vi "HRTF_SynchronizedMeasurement.vi"() -> ()   [LabVIEW 2017]
uses:
  9d5949f9-07ca-45c6-940a-2e3a62ca42df.vi
  <vilib>/express/express analysis/Spectral/Block/exnSpectralBlock spectral measurements RMS poly.vi
  <vilib>/express/express analysis/Spectral/Block/exnSpectralBlock spectral measurements RMS array WFM.vi
  <vilib>/express/express analysis/Spectral/XNode/ExpressSpectralMeasurementsBlockNode.xnode
panel:
  out "current file":dbl
  in  "Number of repetitions (200 is a full revolution)":dbl=200.0
  in  "Rotate stage at COM5":bool=TRUE
  in  "Stim muliplier":dbl=7.0
  in  "4kHz High-pass for stim":bool
  in  "Samples to Read":i32=262144
  in  "Analog Input Sample Clock Source":tag="/Dev1/ao/SampleClock"
  out "Actual Update Generation Rate":dbl=5000.0 format="%0.2f"
  out "Actual Input Rate":dbl=10000.0 format="%0.2f"
  in  "rate":dbl=500000.0 caption="Update Generation Rate" format="%0.2f"
  in  "minimum value":dbl=-10.0 caption="Output Minimum Value" format="%0.2f"
  in  "maximum value":dbl=10.0 caption="Output Maximum Value" format="%0.2f"
  in  "physical channels":tag="Dev1/ao0" caption="Output Physical Channels"
  in  "Maximum Value":dbl=10.0 caption="Input Maximum Value" format="%0.2f"
  in  "Minimum Value":dbl=-10.0 caption="Input Minimum Value" format="%0.2f"
  in  "Rate":dbl=500000.0 caption="Input Rate" format="%0.2f"
  in  "Physical Channel":tag="Dev1/ai0" caption="Input Physical Channel"
  in  "100 Hz high-pass for display":bool
  out "Waveform Graph 2":cluster{"f0":dbl, "df":dbl, "magnitude":dbl[]}[](graph)
  out "Waveform Graph":waveform(dbl)[](graph)
  # "Multiplier was 7 for HRTF measurements.\n4 kHz filter was off for the initial measurement, but it should not affect\nthe response in high frequency.\nIt may not work with 7 V stim."
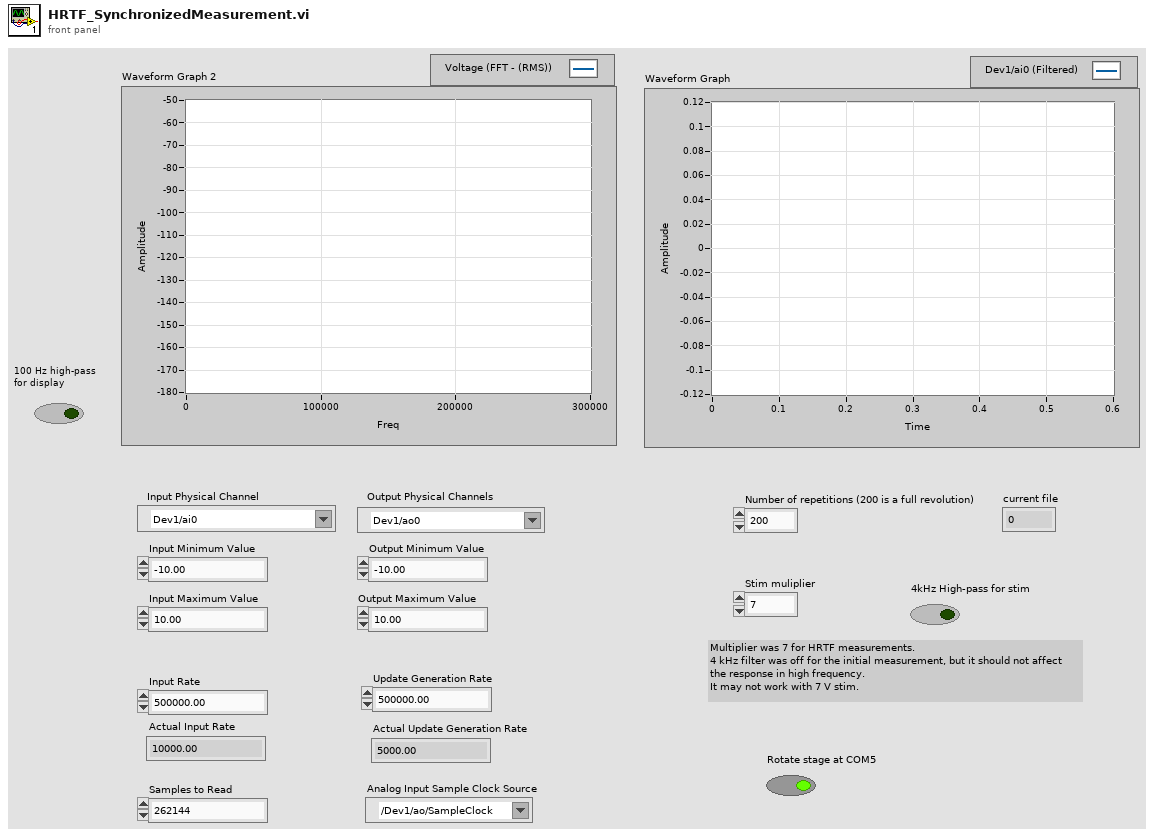
[diagram p1: front panel]
types:
  T1 = cluster{"averaging mode":u16, "weighting mode":u16, "number of averages":u32}
  T2 = cluster{"dB On (F)":bool, "unwrap phase (F)":bool, "convert to degree (F)":bool}
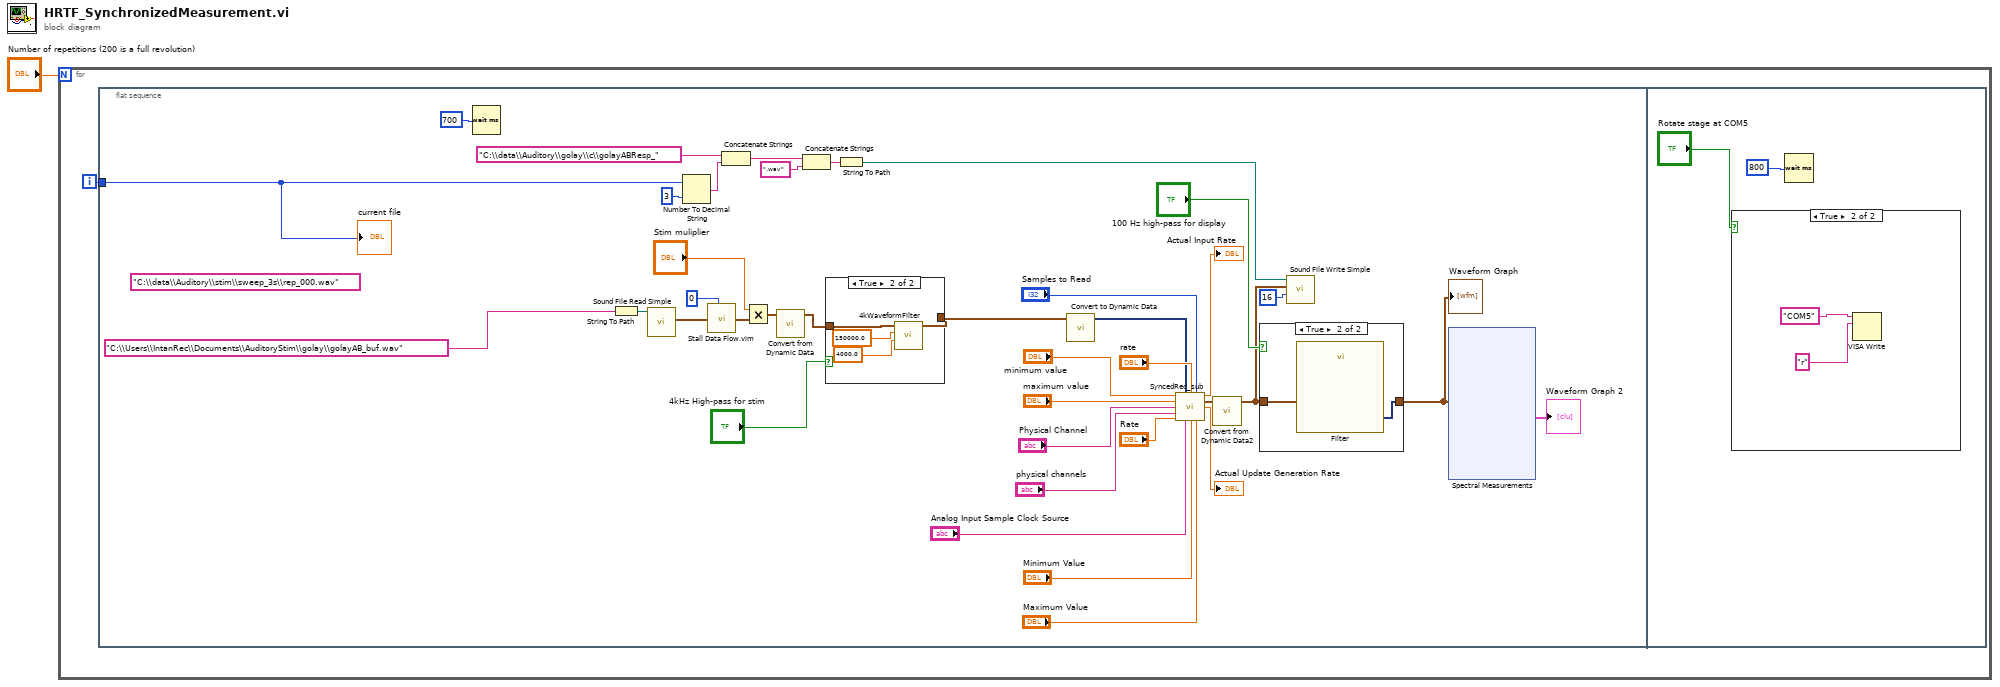
[diagram p0: block diagram]
diagram:
  n1 = for {
    N: "Number of repetitions (200 is a full revolution)" -> [_]
    i -> [w2]
    n2 = flat-sequence {
      tunnel: w2 -> [w3]
      frame #0 {
        (unwired) "C:\\data\\Auditory\\stim\\sweep_3s\\rep_000.wav"
        n3 = Wait (ms)(milliseconds to wait=700) -> ()  [unwired: 1 out]
        n4 = String To Path(string="C:\\Users\\IntanRec\\Documents\\AuditoryStim\\golay\\golayAB_buf.wav") -> (path=w31:path)
        n5 = call <vilib>:"Sound File Read Simple.vi"("path"=w31) -> ("data"=w29:waveform(dbl)[])  [unwired: 7 in, 3 out]
        n6 = Number To Decimal String(number=w3, width (-)=3) -> (decimal integer string=w35:string)
        n7 = call "Stall Data Flow.vim"("value in"=w29, "milliseconds to wait"=0) -> ("value out"=w25:waveform(dbl)[])  [unwired: 1 out]
        n8 = Concatenate Strings("C:\\data\\Auditory\\golay\\c\\golayABResp_", w35) -> (w34:string)
        n9 = Multiply(x="Stim muliplier", y=w25) -> (x*y=w11:waveform(dbl)[])
        n10 = call "Convert from Dynamic Data"("Dynamic Data Type"=w11) -> ("Waveform"=w10:waveform(dbl))  [unwired: 3 in]
        n11 = Concatenate Strings(w34, ".wav") -> (w32:string)
        n12 = case shown="True" "4kHz High-pass for stim" {
          tunnel: w10 -> [w41 w45]
          tunnel: [w41 w44] -> w7
          frame False {
          }
          frame True {
            n13 = call "4kWaveformFilter.vi"("Low cutoff"=4000.0, "High cutoff"=150000.0, "data"=w45) -> ("Waveform"=w44:waveform(dbl))  [unwired: 8 in]
          }
        }
        n14 = String To Path(string=w32) -> (path=w38:path)
        n15 = call "Convert to Dynamic Data"("Waveform"=w7) -> ("Dynamic Data Type"=w12:dynamicdata)  [unwired: 3 in]
        n16 = call "SyncedRec_sub.vi"("minimum value"="minimum value", "signal in"=w12, "rate"="rate", "Samples to Read"="Samples to Read", "maximum value"="maximum value", "Physical Channel"="Physical Channel", "physical channels"="physical channels", "Rate"="Rate", "Analog Input Sample Clock Source"="Analog Input Sample Clock Source", "Minimum Value"="Minimum Value", "Maximum Value"="Maximum Value") -> ("Actual Input Rate"=→"Actual Input Rate":dbl, "data"=w9:waveform(dbl), "Actual Update Generation Rate"=→"Actual Update Generation Rate":dbl)  [unwired: 2 in]
        n17 = call "Convert from Dynamic Data2"("Dynamic Data Type"=w9) -> ("Array of Waveform"=w8:waveform(dbl)[])  [unwired: 3 in]
        n18 = case shown="True" "100 Hz high-pass for display" {
          tunnel: w8 -> [w46 w48]
          tunnel: [w46 w47] -> w27
          frame False {
          }
          frame True {
            n19 = call "Filter"("Signal"=w48) -> ("Filtered Signal"=w47:dynamicdata)  [unwired: 9 in, 1 out]
          }
        }
        "Waveform Graph" <- w27
        n20 = call <vilib>:"Sound File Write Simple.vi"("bits per sample"=16, "data"=w8, "path"=w38) -> ()  [unwired: 7 in, 2 out]
        n21 = xnode "Spectral Measurements"("Signals"=w27) -> ("FFT - (RMS)"=→"Waveform Graph 2":cluster{"f0":dbl, "df":dbl, "magnitude":dbl[]}[])  [unwired: 1 in, 2 out]
        "current file" <- w3
      }
      frame #1 {
        n22 = case shown="True" "Rotate stage at COM5" {
          frame False {
          }
          frame True {
            n23 = VISA Write(VISA resource name="COM5", write buffer="r") -> ()  [unwired: 1 in, 3 out]
          }
        }
        n24 = Wait (ms)(milliseconds to wait=800) -> ()  [unwired: 1 out]
      }
    }
  }
